vi "Stop Core.vi"(10 "final error code":i32, 11 "Event Source In":refnum<class "Chat Window UI Controller.lvclass">) -> (3 "Event Source Out":refnum<class "Chat Window UI Controller.lvclass">)   [LabVIEW 2020, in "Chat Window UI Controller.lvlib" / "Chat Window UI Controller.lvclass"]
doc: "(<B>Filename</B>: Actor Framework.lvlib:Actor.lvclass:Stop Core.vi)\n\nDefines what the actor does before it stops. Use the <B>final error code</B> input to determine whether the actor shut down in response to an error.\n\nBy default, this method does nothing. A descendant class may override it to define behavior, such as shutting down any processes the actor initiated in its override of the Actor Core method."
uses:
  Chat Window UI Controller.lvclass
  C:/Program Files/National Instruments/LabVIEW 2020/vi.lib/ActorFramework/Actor/Actor.lvclass
  <vilib>/ActorFramework/Actor/Actor.lvclass/Actor.ctl
  SubPanel-Actor-Framework-master/Event-Source-Actor/Source/Template Source/Event Source Actor/Event Source Actor.lvclass
  <vilib>/ActorFramework/Actor/Actor.lvclass
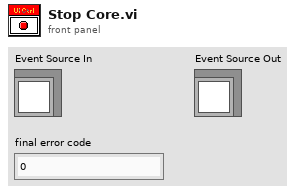
[diagram p1: front panel]
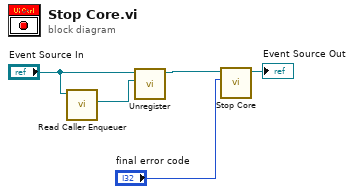
[diagram p0: block diagram]
diagram:
  n1 = call <vilib>:"Read Caller Enqueuer.vi"("Actor"="Event Source In") -> ("Caller Enqueuer"=w1:refnum<class "Message Enqueuer.lvclass">)  [unwired: 10 in]
  n2 = call-dynamic "Unregister.vi"("Registrant Enq"=w1, "Event Source In"="Event Source In") -> ("Event Source Out"=w3:refnum<class "Chat Window UI Controller.lvclass">)  [unwired: 8 in, 1 out]
  n3 = call-parent "Stop Core.vi"("final error code"="final error code", "Event Source In"=w3) -> ("Event Source Out"=→"Event Source Out":refnum<class "Chat Window UI Controller.lvclass">)  [unwired: 9 in]
